vi "Listen.vi"(8 "error in (no error)":errorcluster, 11 "Debug Message Receiver in":refnum<class "Mock Debug Message Receiver.lvclass">) -> (0 "error out":errorcluster, 3 "Debug Message Receiver out":refnum<class "Mock Debug Message Receiver.lvclass">)   [LabVIEW 2020]
uses:
  Process/Debug Process.lvclass
  Mock Debug Message Receiver.lvclass
  C:/Users/anton/Documents/GitHub/triarc-debugger/source/Process/Debug Process.lvclass
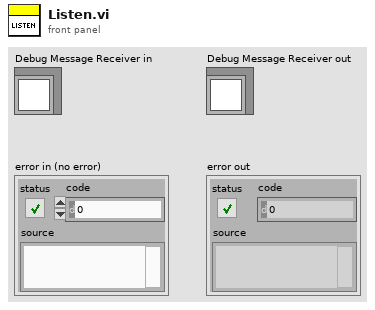
[diagram p1: front panel]
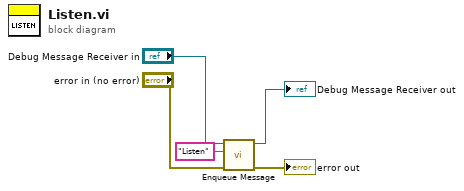
[diagram p0: block diagram]
diagram:
  n1 = call "Enqueue Message.vi"("error in (no error)"="error in (no error)", "Message"="Listen", "Process In"="Debug Message Receiver in") -> ("error out"=→"error out":errorcluster, "Process Out"=→"Debug Message Receiver out":refnum<class "Mock Debug Message Receiver.lvclass">)  [unwired: 7 in]
